vi "Acquisition & Generation (with  Snapshot) RT Test.vi"() -> ()   [LabVIEW 2014]
uses:
  <vilib>/rvi/interface/nirviOpenFPGA/nirviOpenFPGA.xnode
  <vilib>/rvi/interface/nirviMethod/nirviMethod.xnode
  <vilib>/FPGAPlugInAG/Dynamic/niLvFpga_Run_Dynamic.vi
  <vilib>/rvi/interface/nirviReadWriteControl/nirviReadWriteControl.xnode
  <vilib>/rvi/interface/Simulation/niFpgaSimulationCallBeginRW.vi
  <vilib>/rvi/errors/niLvFpgaAdjustHostInterfaceError.vi
  <vilib>/FPGAPlugInAG/Dynamic/niLvFpga_ConfigureFifo_Dynamic.vi
  <vilib>/rvi/errors/niLvFpgaMergeErrorWithErrorCode.vi
  <vilib>/FPGAPlugInAG/Dynamic/niLvFpga_StartFifo_Dynamic.vi
  <vilib>/FPGAPlugInAG/Dynamic/niLvFpga_Abort_Dynamic.vi
  <vilib>/rvi/interface/nirviCloseFPGA/nirviCloseFPGA.xnode
  <vilib>/FPGAPlugInAG/Dynamic/niLvFpga_ReadFifo_Dynamic.vi
  <vilib>/Platform/TimedLoop/XDataNode/wakeup.ctl
  <vilib>/Platform/TimedLoop/XDataNode/XDNodeRunTimeDep.lvlib
  <vilib>/Platform/TimedLoop/XDataNode/nitl_modes.ctl
  <vilib>/Platform/TimedLoop/XDataNode/timing_clust.ctl
  <vilib>/Platform/TimedLoop/XDataNode/XDataNode.xnode
  FPGA Target/Test VIs/Acqusition & Generation (with Snapshot) test.vi
  NiFpgaLv.dll
  <vilib>/Utility/error.llb/Error Cluster From Error Code.vi
  <vilib>/FPGAPlugInAG/Dynamic/niLvFpga_Close_Dynamic.vi
panel:
  out "Modulation Signal":dbl[](graph)
  out "Signal":dbl[](graph)
  in  "stop":bool
  in  "Snapshot":bool
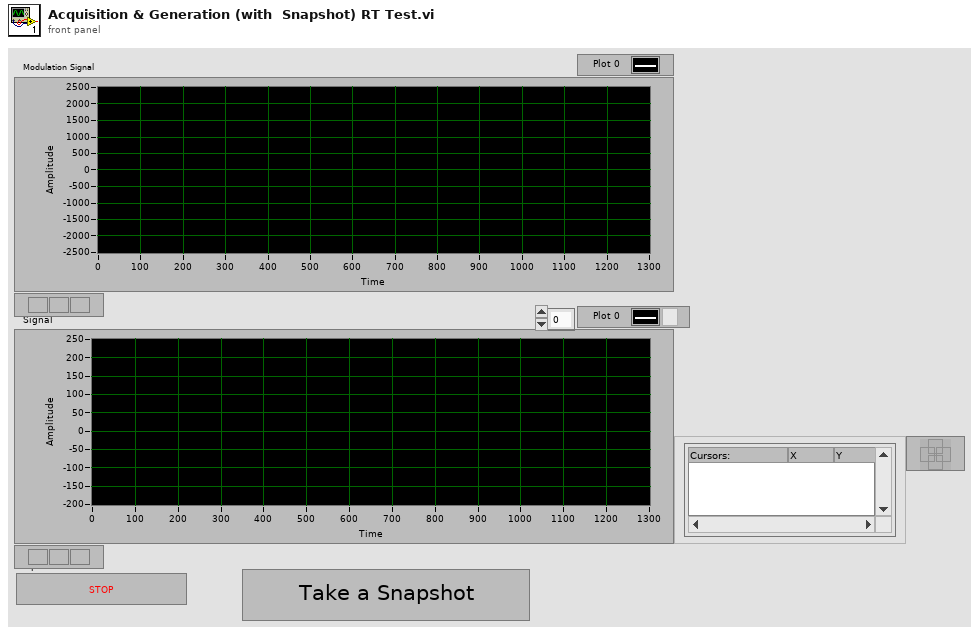
[diagram p1: front panel]
types:
  T1 = typedef "XDNodeRunTimeDep.lvlib/timing_clust.ctl" = cluster{"Expected End [f-1]":u64, "Actual End [f-1]":u64, "Finished Late? [f-1]":bool, "Expected End [i-1]":u64, "Actual End [i-1]":u64, "Finished Late? [i-1]":bool, "Expected Start [i]":u64, "Actual Start [i]":u64, "Expected Start [f]":u64, "Actual Start [f]":u64, "Source Name":string, "Structure Name":string, "Period":i64, "Deadline":i64, "Offset":i64, "Start":i64, "Priority":i32, "Timeout":i32, "Mode":T2, "Wakeup Reason":T3, "Error":errorcluster, "Source Type":string, "Secondary Source Type":string, "Global End Time":u64, "Global Start Time":u64, "Frame Duration":u64, "Iteration Duration":u64, "Assigned CPU":i32, "I/O Scan Engine Mode":u32}
  T2 = typedef "XDNodeRunTimeDep.lvlib/nitl_modes.ctl" = enum32{"No Change", "Process missed periods, maintain original phase", "Discard missed periods, maintain original phase", "Process missed periods, ignore original phase", "Discard missed periods, ignore original phase"}
  T3 = typedef "XDNodeRunTimeDep.lvlib/wakeup.ctl" = enum32{"Normal", "Aborted", "Asynchronous wakeup", "Timing source error", "Timed loop error", "Timeout"}
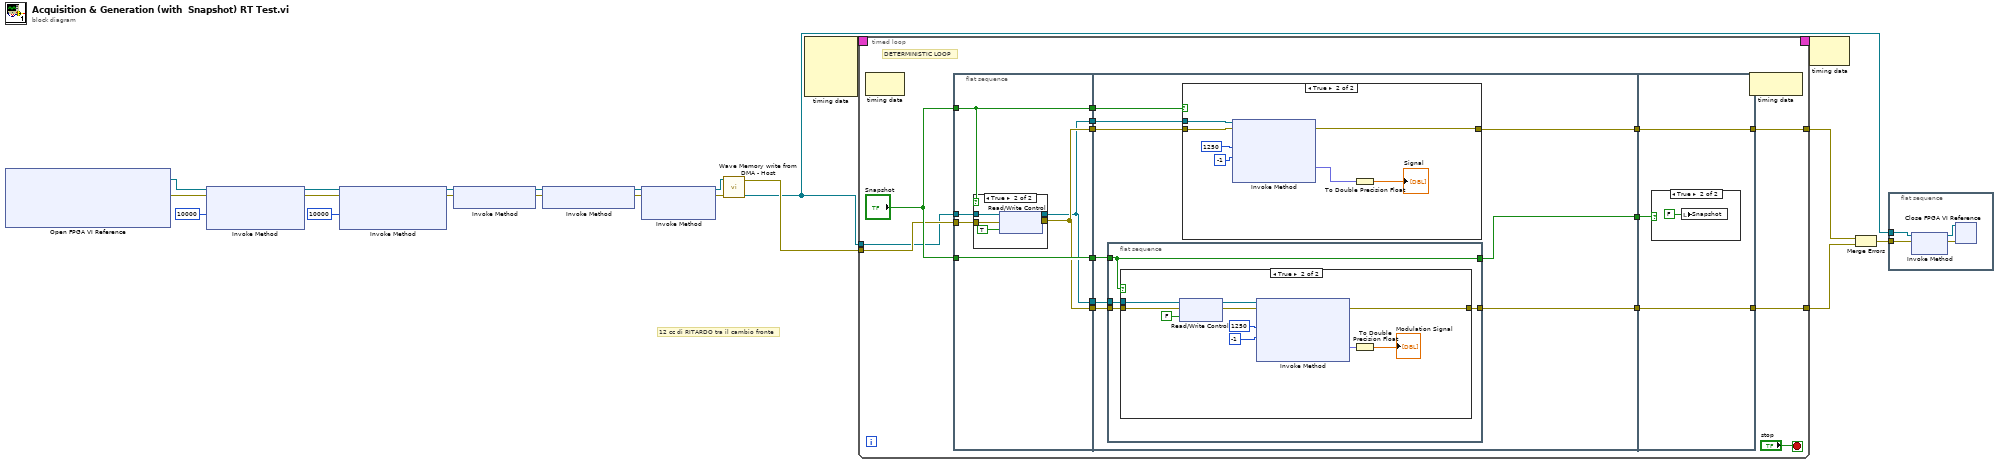
[diagram p0: block diagram]
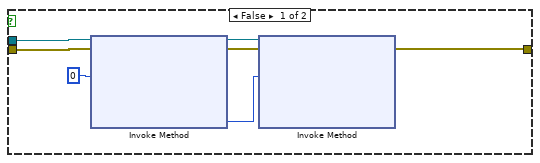
[diagram p3: hidden frame]
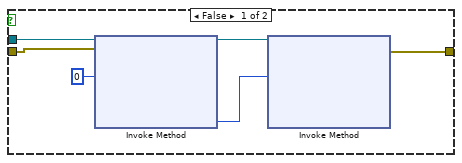
[diagram p4: hidden frame]
diagram:
  # "12 cc di RITARDO tra il cambio fronte"
  n1 = xnode "Open FPGA VI Reference"() -> ("FPGA VI Reference Out"=w8:refnum<k20>, "error out"=w9:errorcluster)  [unwired: 2 in]
  n2 = xnode "Invoke Method"("FPGA VI Reference In"=w8, "error in"=w9, "Requested Depth"=u32 10000) -> ("FPGA VI Reference Out"=w19:refnum<k20>, "error out"=w18:errorcluster)  [unwired: 1 out]
  n3 = xnode "Invoke Method"("FPGA VI Reference In"=w19, "error in"=w18, "Requested Depth"=u32 10000) -> ("FPGA VI Reference Out"=w6:refnum<k20>, "error out"=w7:errorcluster)  [unwired: 1 out]
  n4 = xnode "Invoke Method"("FPGA VI Reference In"=w6, "error in"=w7) -> ("FPGA VI Reference Out"=w15:refnum<k20>, "error out"=w14:errorcluster)
  n5 = xnode "Invoke Method"("FPGA VI Reference In"=w15, "error in"=w14) -> ("FPGA VI Reference Out"=w4:refnum<k20>, "error out"=w5:errorcluster)
  n6 = xnode "Invoke Method"("FPGA VI Reference In"=w4, "error in"=w5) -> ("FPGA VI Reference Out"=w12:refnum<k20>, "error out"=w11:errorcluster)  [unwired: 1 in]
  n7 = call "Wave Memory write from DMA - Host.vi"("error in"=w11, "FPGA VI Reference In"=w12) -> ("FPGA VI Reference Out"=w1:refnum<k20>, "error out"=w3:errorcluster)  [unwired: 7 in, 1 out]
  n8 = node-c288() -> (w21:T1)  [unwired: 4 in]
  n9 = timed-loop {
    tunnel: w1 -> [w32]
    tunnel: w3 -> [w33]
    tunnel: [w35] -> w2
    tunnel: [w36] -> w10
    timing: w21 -> [_]
    timing-out: [_] -> w20
    stop <- "stop" stop-if-true
    # "DETERMINISTIC LOOP"
    n10 = node-c288() -> ()  [unwired: 1 in, 1 out]
    n11 = flat-sequence {
      tunnel: w32 -> [w41]
      tunnel: w33 -> [w42]
      tunnel: "Snapshot" -> [w39]
      tunnel: "Snapshot" -> [w44]
      tunnel: [w43] -> w31
      tunnel: [w44] -> w30
      tunnel: [w39] -> w29
      tunnel: [w43] -> w28
      tunnel: [w40] -> w27
      tunnel: [w40] -> w26
      tunnel: w31 -> [w59]
      tunnel: w30 -> [w54]
      tunnel: w29 -> [w57]
      tunnel: w28 -> [w56]
      tunnel: w27 -> [w55]
      tunnel: w26 -> [w60]
      tunnel: [w58] -> w25
      tunnel: [w52] -> w24
      tunnel: [w53] -> w23
      tunnel: [w97] -> w35
      tunnel: [w98] -> w36
      tunnel: w25 -> [w98]
      tunnel: w24 -> [w97]
      tunnel: w23 -> [w96]
      frame #0 {
        n12 = case shown="True" w39 {
          tunnel: [w45 w50] -> w43
          tunnel: w42 -> [w45 w49]
          tunnel: w41 -> [w46 w48]
          tunnel: [w46 w47] -> w40
          frame False {
          }
          frame True {
            n13 = xnode "Read/Write Control"("FPGA VI Reference In"=w48, "error in"=w49, "Snapshot"=TRUE ("snapshot")) -> ("FPGA VI Reference Out"=w47:refnum<k20>, "error out"=w50:errorcluster)
          }
        }
      }
      frame #1 {
        n14 = flat-sequence {
          tunnel: w60 -> [w64]
          tunnel: w59 -> [w63]
          tunnel: w54 -> [w62]
          tunnel: [w62] -> w53
          tunnel: [w61] -> w52
          frame #0 {
            n15 = case shown="True" w62 {
              tunnel: w64 -> [w71 w74]
              tunnel: w63 -> [w69 w76]
              tunnel: [w68 w80] -> w61
              frame False {
                n16 = xnode "Invoke Method"("FPGA VI Reference In"=w71, "error in"=w69, "Number of Elements"=u32 0) -> ("FPGA VI Reference Out"=w67:refnum<k20>, "error out"=w66:errorcluster, "Elements Remaining"=w70:u32)  [unwired: 1 in, 1 out]
                n17 = xnode "Invoke Method"("FPGA VI Reference In"=w67, "error in"=w66, "Number of Elements"=w70) -> ("FPGA VI Reference Out"=w65:refnum<k20>, "error out"=w68:errorcluster)  [unwired: 1 in, 2 out]
              }
              frame True {
                n18 = xnode "Read/Write Control"("FPGA VI Reference In"=w74, "error in"=w76, "Snapshot"=FALSE ("snapshot")) -> ("FPGA VI Reference Out"=w73:refnum<k20>, "error out"=w75:errorcluster)
                n19 = xnode "Invoke Method"("FPGA VI Reference In"=w73, "error in"=w75, "Number of Elements"=u32 1250, "Timeout (ms)"=-1) -> ("error out"=w80:errorcluster, "Data"=w79:fxp<+/-,12,12>[])  [unwired: 2 out]
                n20 = To Double Precision Float(number=w79) -> (double precision float=→"Modulation Signal":dbl[])
              }
            }
          }
        }
        n21 = case shown="True" w57 {
          tunnel: w55 -> [w87 w91]
          tunnel: w56 -> [w84 w92]
          tunnel: [w83 w95] -> w58
          frame False {
            n22 = xnode "Invoke Method"("FPGA VI Reference In"=w87, "error in"=w84, "Number of Elements"=u32 0) -> ("FPGA VI Reference Out"=w85:refnum<k20>, "Elements Remaining"=w86:u32)  [unwired: 1 in, 2 out]
            n23 = xnode "Invoke Method"("FPGA VI Reference In"=w85, "Number of Elements"=w86) -> ("error out"=w83:errorcluster)  [unwired: 2 in, 3 out]
          }
          frame True {
            n24 = xnode "Invoke Method"("FPGA VI Reference In"=w91, "error in"=w92, "Number of Elements"=u32 1250, "Timeout (ms)"=-1) -> ("error out"=w95:errorcluster, "Data"=w90:fxp<+/-,12,12>[])  [unwired: 2 out]
            n25 = To Double Precision Float(number=w90) -> (double precision float=→"Signal":dbl[])
          }
        }
      }
      frame #2 {
        n26 = case shown="True" w96 {
          frame False {
          }
          frame True {
            n27 = local write "Snapshot"(FALSE ("Snapshot")) -> ()
          }
        }
      }
    }
    n28 = node-c288() -> ()  [unwired: 1 in, 1 out]
  }
  n29 = node-c288(w20) -> ()  [unwired: 1 out]
  n30 = Merge Errors(w10, w2) -> (w13:errorcluster)
  n31 = flat-sequence {
    tunnel: w13 -> [w101]
    tunnel: w1 -> [w100]
    frame #0 {
      n32 = xnode "Invoke Method"("FPGA VI Reference In"=w100, "error in"=w101) -> ("FPGA VI Reference Out"=w102:refnum<k20>, "error out"=w103:errorcluster)
      n33 = xnode "Close FPGA VI Reference"("FPGA VI Reference In"=w102, "error in"=w103) -> ()  [unwired: 1 out]
    }
  }
